vi "PS_Ready.vi"(11 "WaitForReady":bool=TRUE) -> (3 "Ready":bool=TRUE)   [LabVIEW 2014]
uses:
  c_Query_States.ctl
  c_InstructionEnum.ctl
  g_CommandParam.vi
  g_ECS02_Command.vi
panel:
  out "Query Response":string
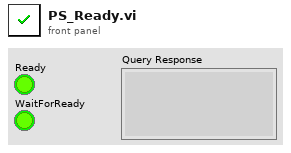
[diagram p1: front panel]
types:
  T1 = typedef "c_Query_States.ctl" = enum16{"Send Query", "Get Response ", "Get Position", "Get Ready Status"}
  T2 = typedef "c_InstructionEnum.ctl" = enum16{"Move Absolute", "Increment", "Move Home", "Motion Kill", "Move Plate", "Set Stepsize", "Query Position"}
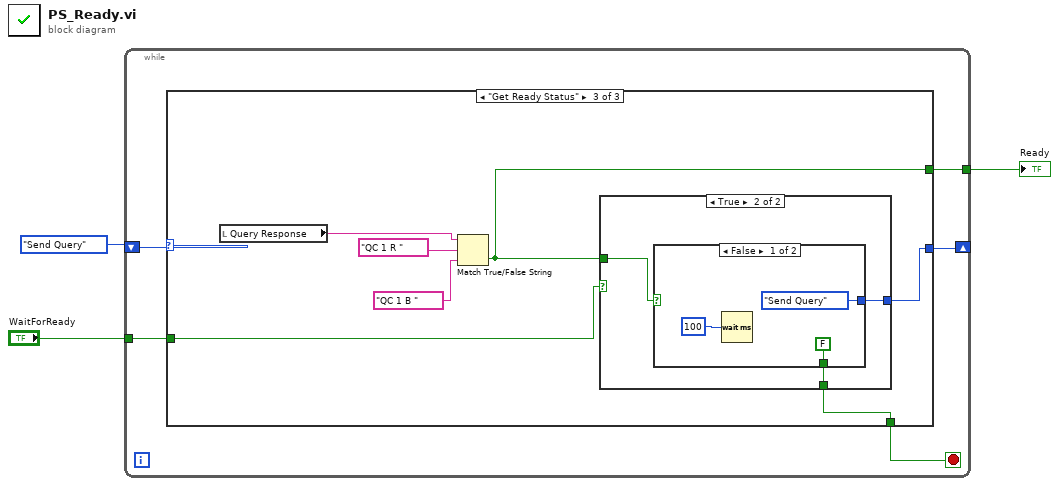
[diagram p0: block diagram]
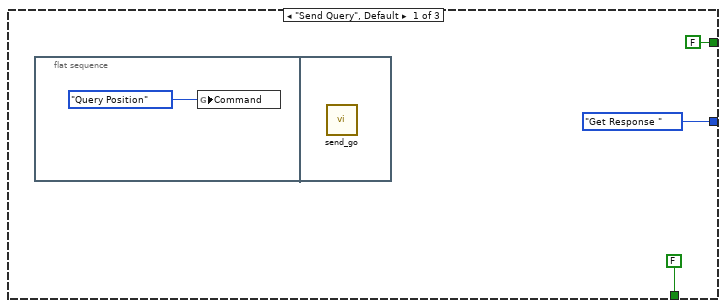
[diagram p2: hidden frame]
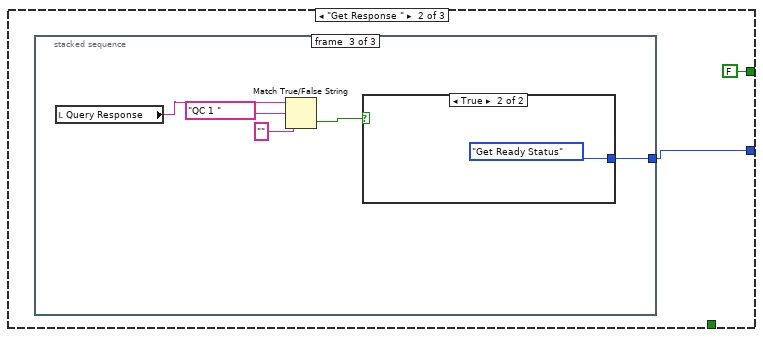
[diagram p3: hidden frame]
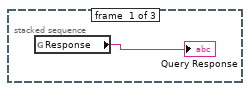
[diagram p4: hidden frame]
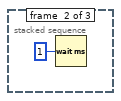
[diagram p5: hidden frame]
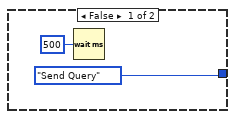
[diagram p6: hidden frame]
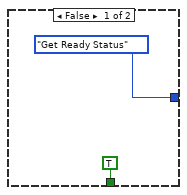
[diagram p7: hidden frame]
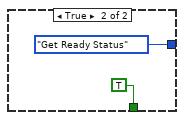
[diagram p8: hidden frame]
diagram:
  n1 = while {
    shift-right: [w7] -> _
    shift-left: c_Query_States."Send Query" -> [w8]
    tunnel: [w5] -> w2
    tunnel: "WaitForReady" -> [w4]
    stop <- w6 stop-if-true
    n2 = case shown="\"Get Ready Status\"" w8 {
      tunnel: [c_Query_States."Get Response " w14 w26] -> w7
      tunnel: [FALSE _ w25] -> w6
      tunnel: [FALSE ("selection") FALSE ("selection") w27] -> w5
      tunnel: w4 -> [_ _ w28]
      frame "Send Query", Default {
        n3 = flat-sequence {
          frame #0 {
            n4 = global write "g_CommandParam.vi" "Command"(c_InstructionEnum."Query Position" ("Command")) -> ()
          }
          frame #1 {
            n5 = call "send_go.vi"() -> ()  [unwired: 12 in]
          }
        }
      }
      frame "Get Response " {
        n6 = stacked-sequence {
          tunnel: [_ _ w19] -> w14
          frame #0 {
            n7 = global read "g_ECS02_Command.vi" "Response"() -> (→"Query Response":string)
          }
          frame #1 {
            n8 = Wait (ms)(milliseconds to wait=u32 1) -> ()  [unwired: 1 out]
          }
          frame #2 {
            n9 = local read "Query Response"() -> (w18:string)
            n10 = Match True/False String(2:"" ("false string"), 3:"QC 1 " ("true string"), 4:w18) -> (0:w17:bool)  [unwired: 1 out]
            n11 = case shown="True" w17 {
              tunnel: [c_Query_States."Send Query" c_Query_States."Get Ready Status"] -> w19
              frame False {
                n12 = Wait (ms)(milliseconds to wait=u32 500) -> ()  [unwired: 1 out]
              }
              frame True {
              }
            }
          }
        }
      }
      frame "Get Ready Status" {
        n13 = local read "Query Response"() -> (w30:string)
        n14 = Match True/False String(2:"QC 1 B " ("true string"), 3:"QC 1 R " ("true string"), 4:w30) -> (0:w27:bool)  [unwired: 1 out]
        n15 = case shown="True" w28 {
          tunnel: w27 -> [_ w36]
          tunnel: [c_Query_States."Get Ready Status" w35] -> w26
          tunnel: [TRUE w34] -> w25
          frame False {
          }
          frame True {
            n16 = case shown="False" w36 {
              tunnel: [c_Query_States."Send Query" c_Query_States."Get Ready Status"] -> w35
              tunnel: [FALSE TRUE] -> w34
              frame False {
                n17 = Wait (ms)(milliseconds to wait=u32 100) -> ()  [unwired: 1 out]
              }
              frame True {
              }
            }
          }
        }
      }
    }
  }
  "Ready" <- w2
